vi "PyLoN_SRS3.vi"() -> ()   [LabVIEW 2014]
uses:
  Labview VIs/PIXIS_TEST/SITK_Labview/Examples70_2_2_0_1/RS Pixis/MaxY.vi
  Labview VIs/PIXIS_TEST/SITK_Labview/Examples70_2_2_0_1/RS Pixis/MaxX.vi
  <vilib>/Utility/file.llb/Write To Spreadsheet File (I64).vi
  <vilib>/Utility/file.llb/Write To Spreadsheet File (DBL).vi
panel:
  in  "stop":bool
  out "error out":errorcluster
  out "Description":string
  out "Increment":dbl
  out "Temperature 2":dbl=-75.0
  in  "error in":errorcluster
  out "x/y":dbl
  in  "CHEK ID":bool
  out "Max Value":dbl
  out "Min Value":dbl
  in  "Param ID":u32
  out "default value":dbl
  out "current value":dbl
  out "num of elements":dbl
  in  "?":bool
  in  "?":T1(tab)
  in  "Shutter State":u16(ring)=2 items=["Always Close", "Open Each Exposure", "Open Until Finish", "Open waiting for triger"]
  in  "Trigger Edge":u16(ring) items=["Positive", "Negative"]
  in  "Timing Mode":u16(ring) items=["Free Run", "Triger First", "Ext Sync", "Bulb Mode", "Variable Mode", "Flash Mode"]
  in  "ADC Speed":u16(ring)=2 items=["ADC Slowest", "ADC Fastest", "Default", "50 kHz", "100 kHz", "200 kHz", "500 kHz", "1 MHz"]
  in  "ADC Gain":u16(ring) items=["ADC Low", "ADC High"]
  in  "Temperature":dbl=-100.0 caption="SET Temperature" format="%.2f"
  in  "Skip Serial  Reg Clean":dbl=1.0 format="%.2f"
  in  "Vertical Timing":dbl=3.2
  out "Vertical Timing":dbl
  in  "Readout Port":i32=4 min=-1 step=1
  in  "?":T2={"X start"=0, "X end"=1023, "X Binning/Grouping"=1, "Y start"=0, "Y end"=1, "Y Binning/Grouping"=1}
  in  "Logic Out":u16(ring) items=["Not Scan", "Shutter", "Not Rady", "Logic 0", "Clearing", "Not Ft Image Shift", "Reserved", "Logic1", "Expos Prog", "Expos", "Image Shift", "Readout", "Acquiring", "Wait For Trig"]
  in  "Use Custom Timing":bool
  out "Readout Time":dbl caption="Readout time (ms)" format="%.2f"
  in  "Temp_bypass":bool
  in  "?":bool
  in  "Exposure Time (s)":dbl=0.004 min=0.0 step=0.001 format="%.3f"
  in  "?":bool
  in  "?":bool
  out "?":u16[](graph)
  in  "file path":path
  in  "File_name":string
  in  "# of spectrum per frame":i32
  in  "# of Frames":i32
  in  "FLIP SPECTRA":bool
  in  "?":bool
  in  "?":bool
  in  "?":bool
  out "?":dbl[](graph)
  in  "?":bool
  in  "Number of Images":u32=1 min=1 step=1
  out "?":dbl[](graph)
  in  "?":bool
  in  "# of Sets":i32
  out "Current Set":u32=24
  in  "#Ground per set":u32=3
  in  "Timepoints":dbl[](array[numeric])=[200.0, 100.0, 300.0, 400.0, 500.0]
  in  "File Path":path
  in  "File Name":string
  in  "Ground State\nSubstract?":bool
  in  "PyLonN Error In":errorcluster
  out "PyLoN Error Out":errorcluster
  out "PyLoN Ready":bool
  out "PyLoN \nTemperature":dbl
  # "REGION OF INTEREST"
  # "TRIGGER"
  # "ADC"
  # "SHUTTER"
  # "INPUT VARIABLES"
  # "TTL LOGIC"
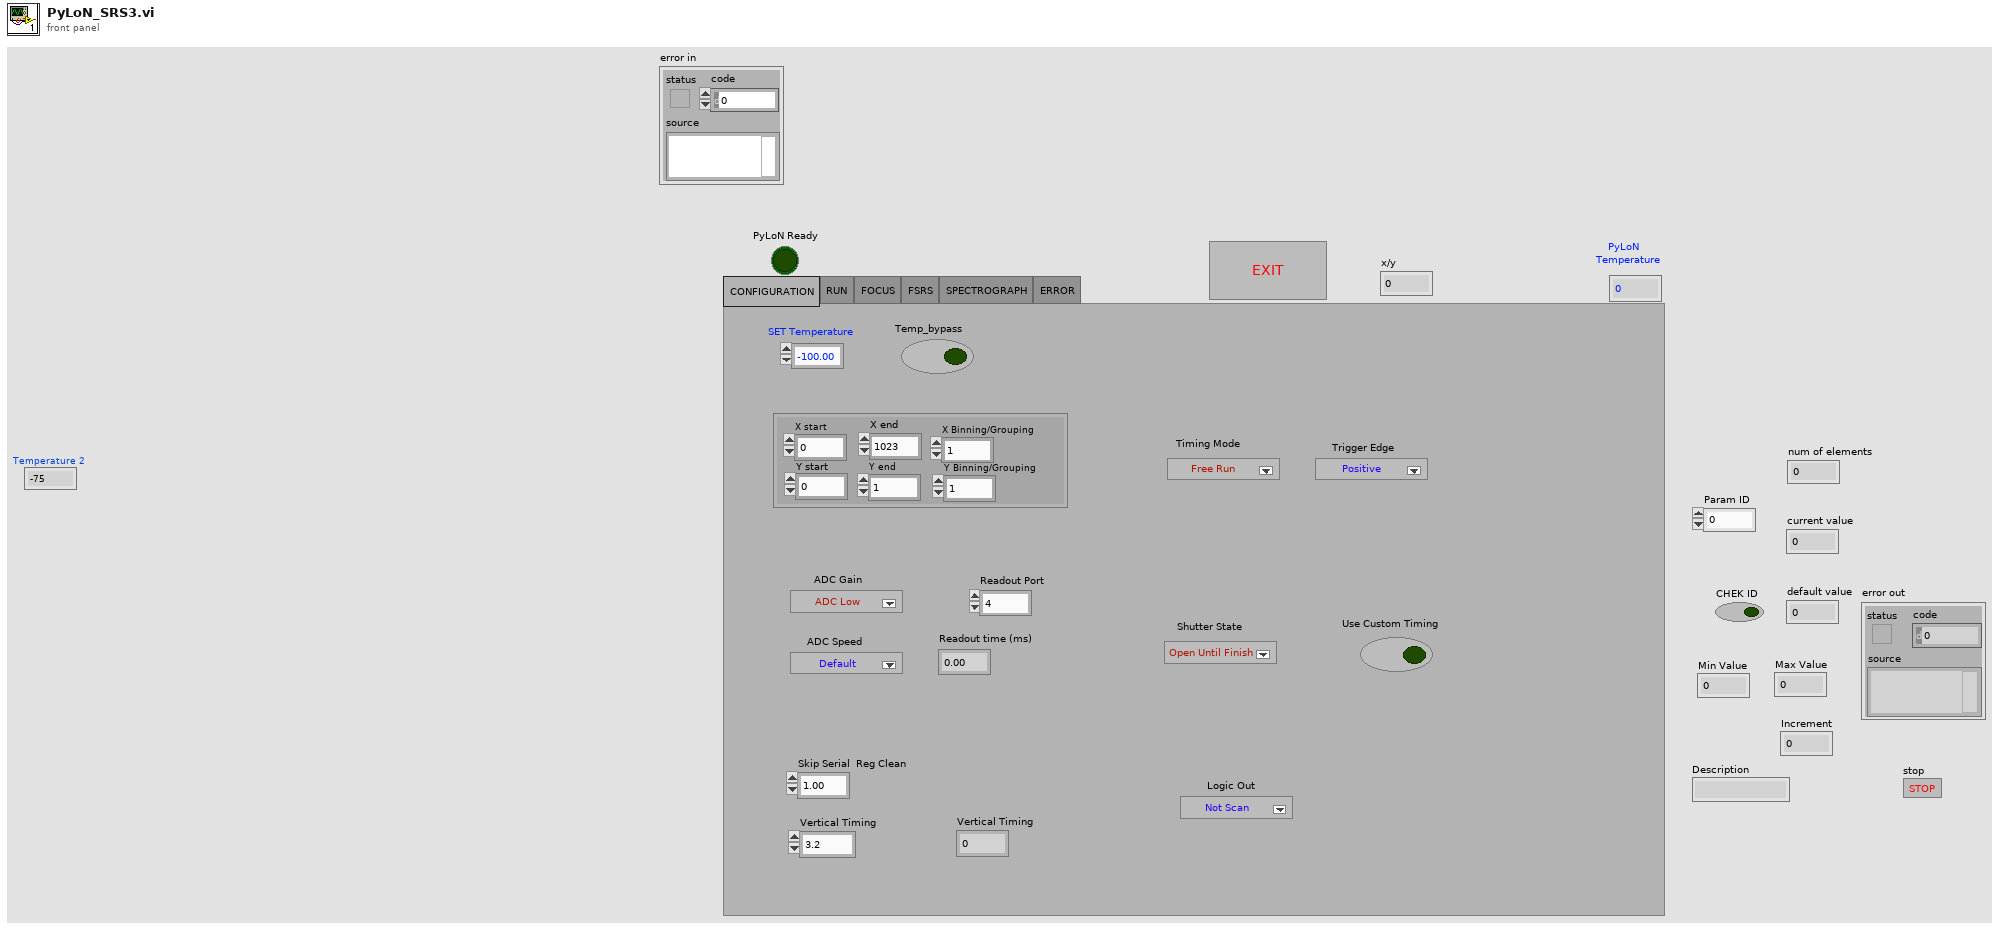
[diagram p1: front panel]
types:
  T1 = enum32{"CONFIGURATION", "RUN", "FOCUS", "FSRS", "SPECTROGRAPH", "ERROR"}
  T2 = cluster{"X start":u32, "X end":u32, "X Binning/Grouping":u32, "Y start":u32, "Y end":u32, "Y Binning/Grouping":u32}
  T3 = enum32{"Initializing", "RUN", "FSRS", "Monochromator", "Errors"}
  T4 = cluster{"Param ID":u32, "Avail Flag":u8, "Current Value":dbl, "Default Value":dbl, "Min Value":dbl, "Max Value":dbl, "Increment":dbl, "Data Type":u32, "Access Type":u32, "Bit Used Flag":u32, "Number of Enums":u32, "Description":string}
  T5 = cluster{"acquire focus mode":u32, "Exposure Time (s)":dbl, i32, "Software accumulation":u32}
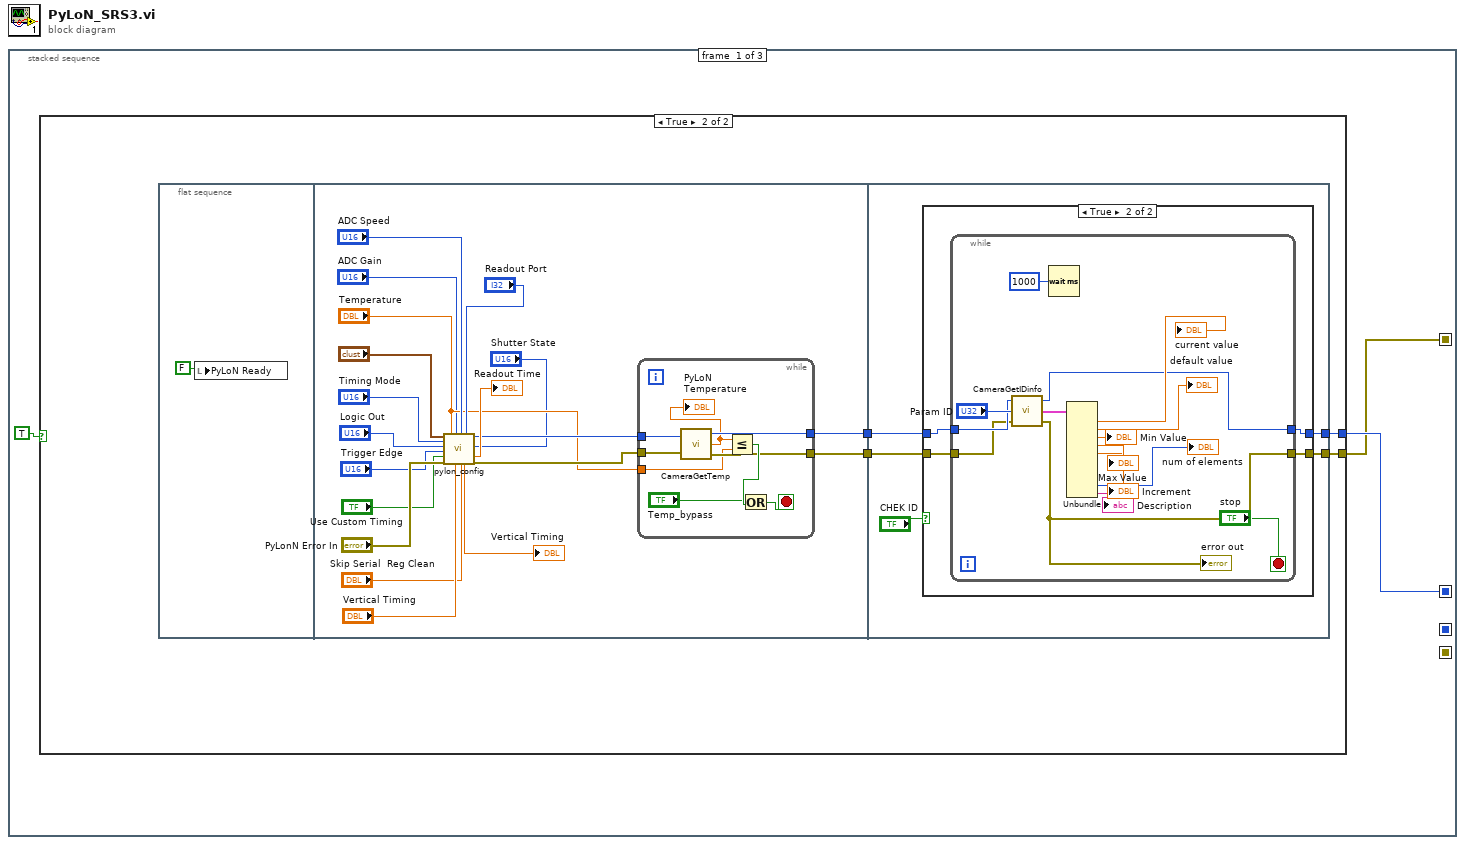
[diagram p0: block diagram]
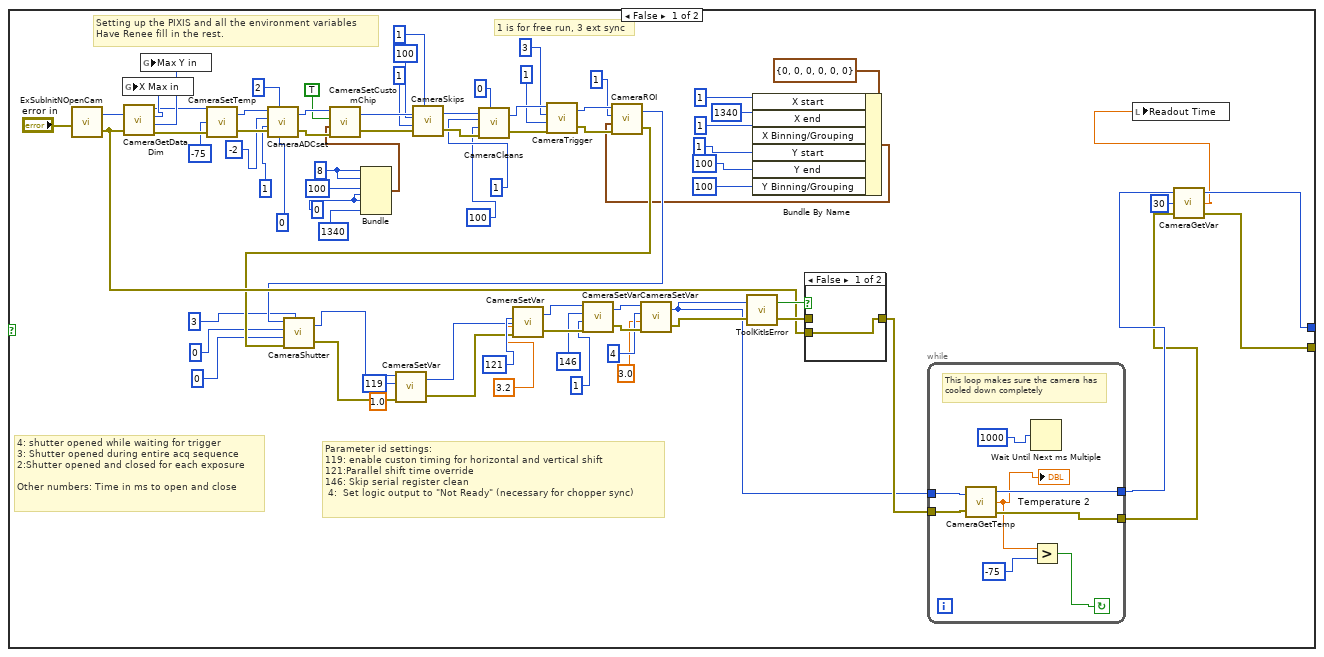
[diagram p2: hidden frame]
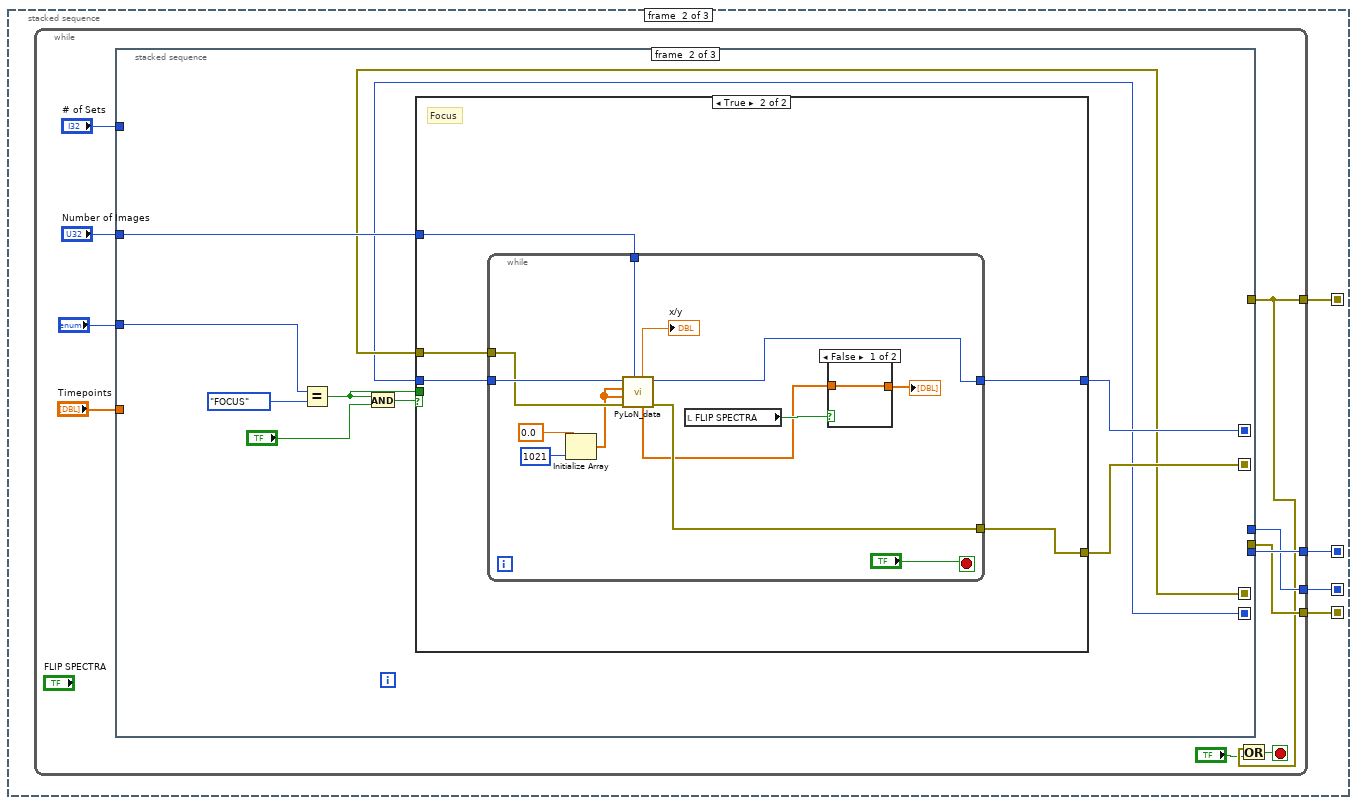
[diagram p5: hidden frame]
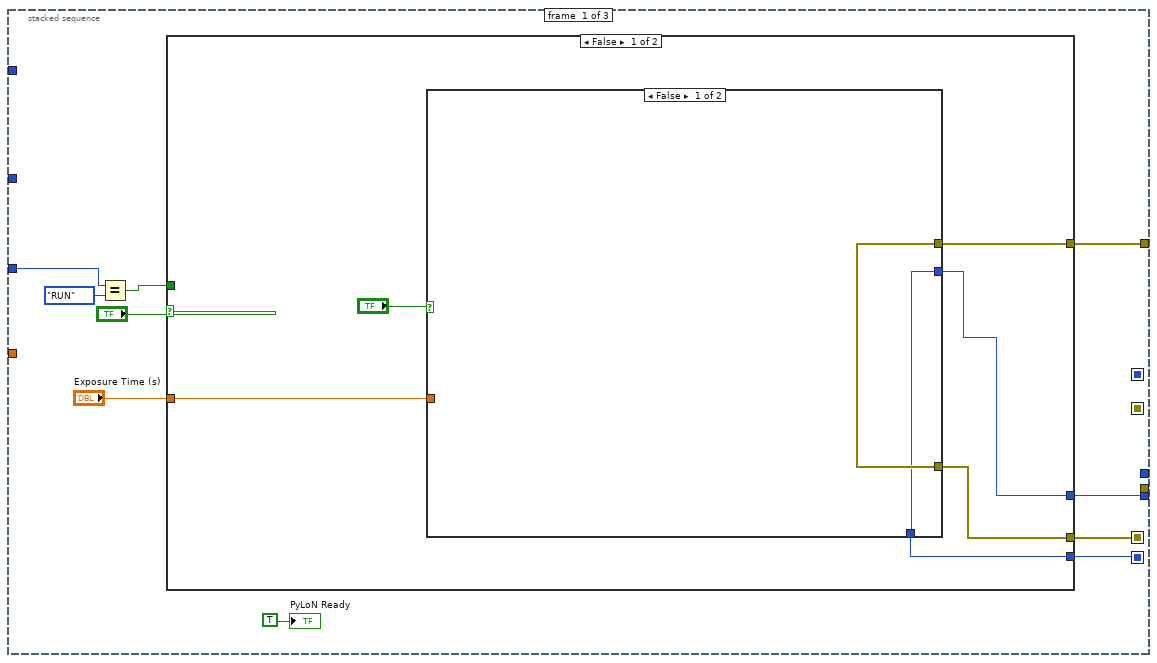
[diagram p6: hidden frame]
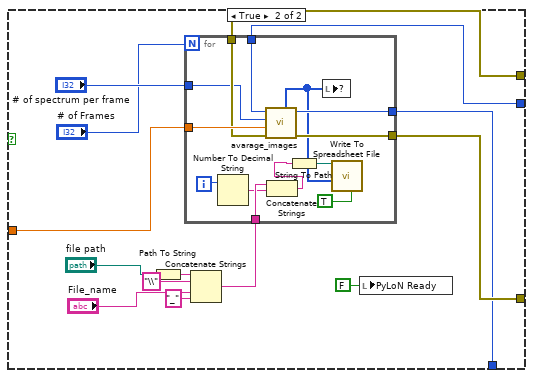
[diagram p7: hidden frame]
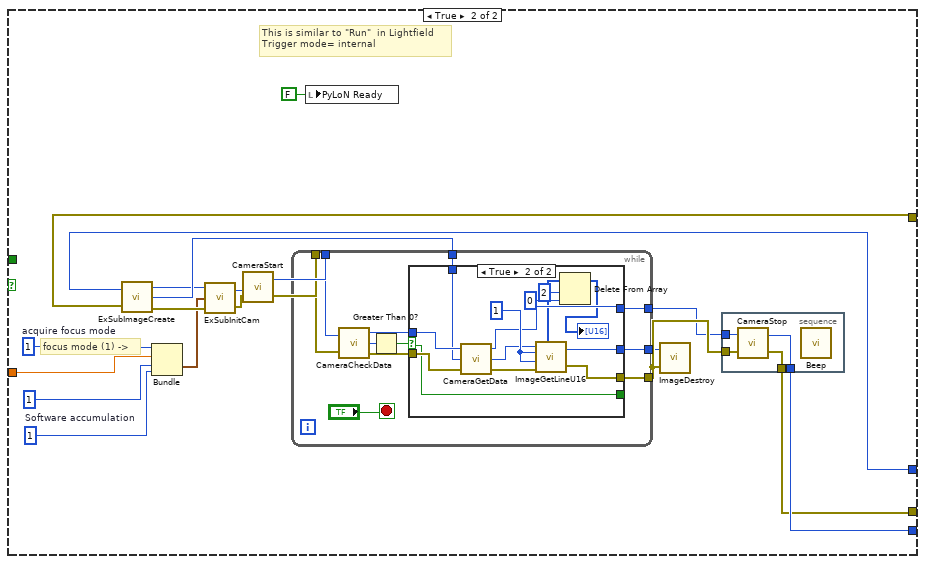
[diagram p8: hidden frame]
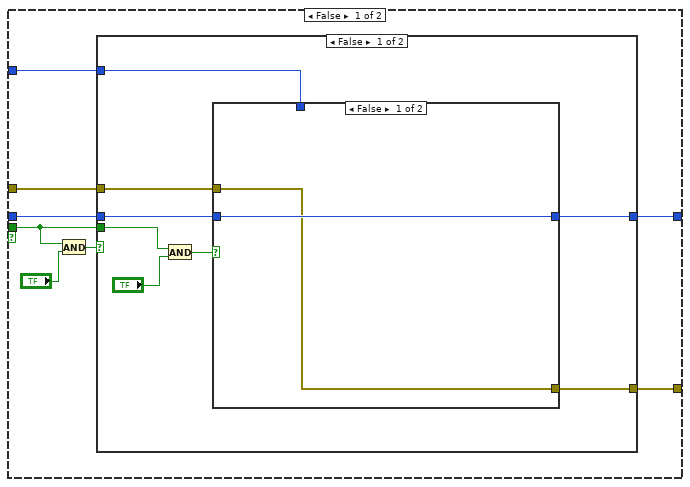
[diagram p10: hidden frame]
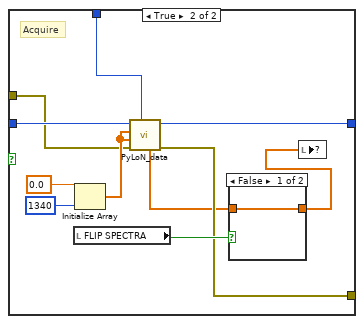
[diagram p11: hidden frame]
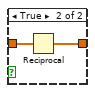
[diagram p12: hidden frame]
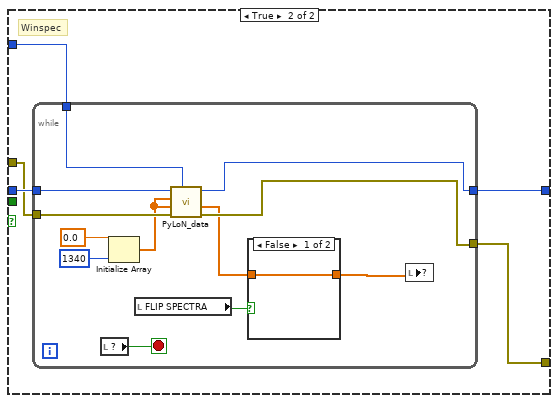
[diagram p13: hidden frame]
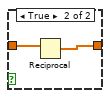
[diagram p14: hidden frame]
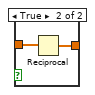
[diagram p15: hidden frame]
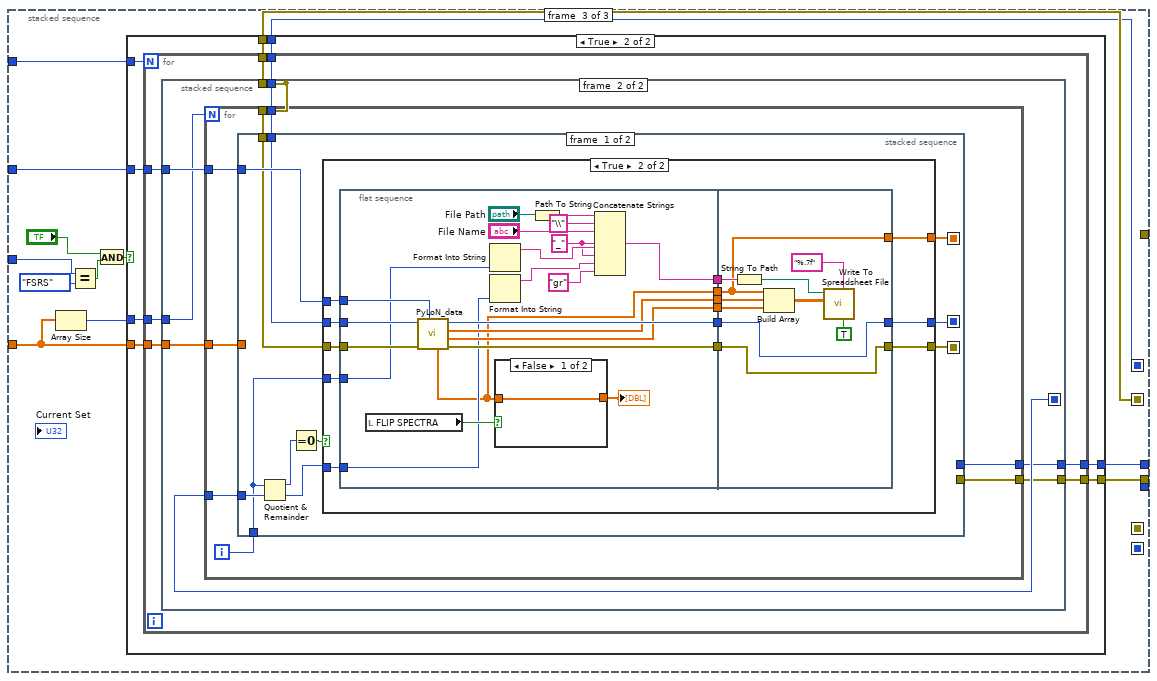
[diagram p16: hidden frame]
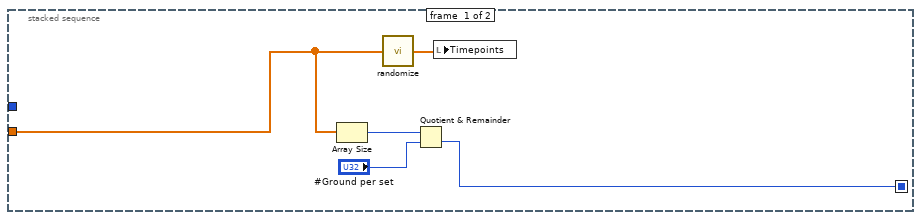
[diagram p18: hidden frame]
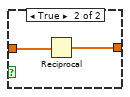
[diagram p20: hidden frame]
diagram:
  n1 = stacked-sequence {
    seq-local: [w1 _ _] -> [_ w152 _]
    seq-local: [w3 _ _] -> [_ w155 _]
    seq-local: [_ w154 _] -> [_ _ w517]
    seq-local: [_ w153 _] -> [_ _ w516]
    frame #0 {
      n2 = case shown="True" TRUE {
        tunnel: [w21 w94] -> w3
        tunnel: [w22 w93] -> w1
        frame False {
          w66 = 0
          w68 = 8
          # "4: shutter opened while waiting for trigger\n3: Shutter opened during entire acq sequence\n2:Shutter opened and closed for each exposure\n\nOther numbers: Time in ms to open and close"
          # "1 is for free run, 3 ext sync"
          # "Parameter id settings:\n119: enable custon timing for horizontal and vertical shift\n121:Parallel shift time override\n146: Skip serial register clean\n 4:  Set logic output to \"Not Ready\" (necessary for chopper sync)"
          # "Setting up the PIXIS and all the environment variables\nHave Renee fill in the rest."
          n3 = call "ExSubInitNOpenCam.vi"("error in (no error)"="error in") -> ("Camera Handle"=w81:u32, "error out"=w46:errorcluster)
          n4 = call <userlib>:"CameraGetDataDim.vi"("Camera Handle"=w81, "error in"=w46) -> ("Camera Handle"=w78:u32, "Xdim"=w80:u32, "Ydim"=w79:u32, "error out"=w77:errorcluster)
          n5 = global write "MaxX.vi" "X Max in"(w80) -> ()
          n6 = global write "MaxY.vi" "Max Y in"(w79) -> ()
          n7 = call <userlib>:"CameraSetTemp.vi"("error in (no error)"=w77, "Temperature"=-75, "Camera Handle"=w78) -> ("error out"=w74:errorcluster, "Camera Handle"=w75:u32)
          n8 = call <userlib>:"CameraADCset.vi"("ADC offset"=0, "Read Out port"=2, "error in (no error)"=w74, "ADC Gain"=1, "ADC Speed"=-2, "Camera Handle"=w75) -> ("error out"=w69:errorcluster, "Camera Handle"=w70:u32)
          n9 = Bundle(w68, w68, 100, w66, w66, 1340) -> (w64:cluster{i32, i32, i32, i32, i32, i32})  [unwired: 1 in]
          n10 = call <userlib>:"CameraSetCustomChip.vi"("error in (no error)"=w69, "Custom Chip Settings"=w64, "Enable/Disable Custom Chip"=TRUE, "Camera Handle"=w70) -> ("error out"=w61:errorcluster, "Camera Handle"=w62:u32)
          n11 = call <userlib>:"CameraSkips.vi"("Camera Handle"=w62, "Minimum Block Size"=100, "Number of Minimum blocks"=1, "error in"=w61, "Type of Skips"=1) -> ("Camera Handle"=w56:u32, "error out"=w57:errorcluster)
          n12 = call <userlib>:"CameraCleans.vi"("Camera Handle"=w56, "Number of Clears"=1, "Number of Strips Per Clear"=100, "error in"=w57, "Continuous Clears"=0) -> ("Camera Handle"=w51:u32, "error out"=w52:errorcluster)
          n13 = call <userlib>:"CameraTrigger.vi"("error in"=w52, "Trigger Edge"=1, "Timing Mode"=3, "Camera Handle"=w51) -> ("error out"=w38:errorcluster, "Camera Handle"=w37:u32)
          n14 = Bundle By Name(cluster=T2 {"X start"=0, "X end"=0, "X Binning/Grouping"=0, "Y start"=0, "Y end"=0, "Y Binning/Grouping"=0} ("ROI Params"), "X start"=u32 1, "X end"=u32 1340, "X Binning/Grouping"=u32 1, "Y start"=u32 1, "Y end"=u32 100, "Y Binning/Grouping"=u32 100) -> (w28:T2)
          n15 = call <userlib>:"CameraROI.vi"("error in"=w38, "ROI Params"=w28, "ROI Index"=1, "Camera Handle"=w37) -> ("error out"=w34:errorcluster, "Camera Handle"=w33:u32)
          n16 = call <userlib>:"CameraShutter.vi"("Camera Handle"=w33, "Shutter Comp Time: Pre Open"=0, "Shutter Comp Time: Post Open"=0, "error in"=w34, "Shutter State"=3) -> ("Camera Handle"=w9:u32, "error out"=w7:errorcluster)
          n17 = call <userlib>:"CameraSetVar.vi"("error in"=w7, "Value"=1.0, "Parameter ID"=u32 119, "Camera Handle"=w9) -> ("error out"=w6:errorcluster, "CameraHandle"=w8:u32)
          n18 = call <userlib>:"CameraSetVar.vi"("error in"=w6, "Value"=3.2, "Parameter ID"=121, "Camera Handle"=w8) -> ("error out"=w19:errorcluster, "CameraHandle"=w18:u32)
          n19 = call <userlib>:"CameraSetVar.vi"("error in"=w19, "Value"=1, "Parameter ID"=146, "Camera Handle"=w18) -> ("error out"=w14:errorcluster, "CameraHandle"=w13:u32)
          n20 = call <userlib>:"CameraSetVar.vi"("error in"=w14, "Value"=3.0, "Parameter ID"=4, "Camera Handle"=w13) -> ("error out"=w29:errorcluster, "CameraHandle"=w26:u32)
          n21 = call <userlib>:"ToolKitIsError.vi"("error in"=w29, "Reserved"=w26) -> ("error out"=w47:errorcluster, "Error Flag"=w48:bool)
          n22 = case shown="False" w48 {
            tunnel: w47 -> [_ w92]
            tunnel: [w91 w92] -> w27
            tunnel: w46 -> [w91 _]
            frame False {
            }
            frame True {
            }
          }
          n23 = while {
            tunnel: w27 -> [w89]
            tunnel: [w88] -> w23
            tunnel: w26 -> [w87]
            tunnel: [w86] -> w24
            stop <- w84 continue-if-true
            # "This loop makes sure the camera has cooled down completely"
            n24 = call <userlib>:"CameraGetTemp.vi"("Camera Handle"=w87, "error in (no error)"=w89) -> ("Camera Handle"=w86:u32, "Temperature"=w83:dbl, "error out"=w88:errorcluster)
            "Temperature 2" <- w83
            n25 = Wait Until Next ms Multiple(millisecond multiple=1000 ("ADC Gain")) -> ()  [unwired: 1 out]
            n26 = Greater?(x=w83, y=-75) -> (0:w84:bool)
          }
          n27 = call <userlib>:"CameraGetVar.vi"("error in"=w23, "Parameter ID"=u32 30, "Camera Handle"=w24) -> ("error out"=w22:errorcluster, "Value"=w20:dbl, "Camera Handle"=w21:u32)
          n28 = local write "Readout Time"(w20) -> ()
        }
        frame True {
          n29 = flat-sequence {
            tunnel: [w104] -> w96
            tunnel: [w102] -> w95
            tunnel: [w126] -> w93
            tunnel: [w129] -> w94
            tunnel: w96 -> [w130]
            tunnel: w95 -> [w128]
            frame #0 {
              n30 = local write "PyLoN Ready"(FALSE ("PyLoN Ready")) -> ()
            }
            frame #1 {
              n31 = call "pylon_config.vi"(0:"?", "Timing Mode"="Timing Mode", "Logic Out"="Logic Out", "Trigger Edge"="Trigger Edge", "Use Custom Chip"="Use Custom Timing", "PyLonN Error In"="PyLonN Error In", "Temperature"="Temperature", "ADC Gain"="ADC Gain", "Vertical Timing"="Vertical Timing", "ADC Speed"="ADC Speed", "Skip Serial  Reg Clean"="Skip Serial  Reg Clean", "Readout Port"="Readout Port", "Shutter State"="Shutter State") -> ("Vertical Timing"=→"Vertical Timing":dbl, "CameraHandle"=w105:u32, "Readout Time"=→"Readout Time":dbl, "error out"=w103:errorcluster)  [unwired: 3 in]
              n32 = while {
                tunnel: [w125] -> w104
                tunnel: w105 -> [w122]
                tunnel: w103 -> [w121]
                tunnel: [w120] -> w102
                tunnel: "Temperature" -> [w118]
                stop <- w124 stop-if-true
                n33 = call <userlib>:"CameraGetTemp.vi"("Camera Handle"=w122, "error in (no error)"=w121) -> ("Camera Handle"=w125:u32, "Temperature"=w119:dbl, "error out"=w120:errorcluster)
                "PyLoN \nTemperature" <- w119
                n34 = Less Or Equal?(x=w119, y=w118) -> (x <= y?=w123:bool)
                n35 = Or(x="Temp_bypass", y=w123) -> (x .or. y?=w124:bool)
              }
            }
            frame #2 {
              n36 = case shown="True" "CHEK ID" {
                tunnel: w130 -> [w132 w136]
                tunnel: [w132 w135] -> w129
                tunnel: w128 -> [w131 w134]
                tunnel: [w131 w133] -> w126
                frame False {
                }
                frame True {
                  n37 = while {
                    tunnel: w136 -> [w146]
                    tunnel: [w145] -> w135
                    tunnel: w134 -> [w144]
                    tunnel: [w143] -> w133
                    stop <- "stop" stop-if-true
                    n38 = call <userlib>:"CameraGetIDinfo.vi"("error in"=w144, "Param ID"="Param ID", "Camera handle"=w146) -> ("error out"=w143:errorcluster, "Param ID Information"=w151:T4, "Camera handle"=w145:u32)
                    "error out" <- w143
                    n39 = Wait (ms)(milliseconds to wait=u32 1000) -> ()  [unwired: 1 out]
                    n40 = Unbundle(w151) -> ("Current Value"=→"current value":dbl, "Default Value"=→"default value":dbl, "Min Value"=→"Min Value":dbl, "Max Value"=→"Max Value":dbl, "Increment"=→"Increment":dbl, "Number of Enums"=→"num of elements":u32, "Description"=→"Description":string)  [unwired: 5 out]
                  }
                }
              }
            }
          }
        }
      }
    }
    frame #1 {
      n41 = while {
        tunnel: w155 -> [w165]
        tunnel: w152 -> [w157]
        tunnel: [w161] -> w154
        tunnel: [w160] -> w153
        stop <- w158 stop-if-true
        n42 = stacked-sequence {
          seq-local: [_ w268 _] -> [_ _ w353]
          seq-local: [_ w267 _] -> [_ _ w355]
          seq-local: [w170 _ _] -> [_ w265 _]
          seq-local: [w171 _ _] -> [_ w266 _]
          tunnel: w165 -> [w168 _ _]
          tunnel: w157 -> [w175 _ _]
          tunnel: "?" -> [w172 w273 w359]
          tunnel: "Number of Images" -> [_ w271 w356]
          tunnel: "Timepoints" -> [_ _ w348]
          tunnel: [_ _ w352] -> w161
          tunnel: [_ _ w351] -> w160
          tunnel: "# of Sets" -> [_ _ w349]
          frame #0 {
            n43 = Equal?(x=w172, y=T3."RUN") -> (x = y?=w169:bool)
            n44 = case shown="False" "?" {
              tunnel: w175 -> [w181 w213]
              tunnel: [w178 w216] -> w170
              tunnel: [w180 w215] -> w171
              tunnel: w169 -> [_ _]
              tunnel: w168 -> [w179 w214]
              tunnel: "Exposure Time (s)" -> [w177 w211]
              frame False {
                n45 = case shown="False" "?" {
                  tunnel: w181 -> [w183 w195]
                  tunnel: [w183 w194] -> w180
                  tunnel: w179 -> [w182 w196]
                  tunnel: [w182 w193] -> w178
                  tunnel: w177 -> [_ w197]
                  frame False {
                  }
                  frame True {
                    n46 = Path To String(path="file path") -> (string=w189:string)
                    n47 = Concatenate Strings(w189, "\\" ("string"), "File_name", "_" ("string")) -> (w184:string)
                    n48 = for {
                      N: "# of Frames" -> [_]
                      tunnel: w197 -> [w210]
                      tunnel: w196 -> [w209]
                      tunnel: w195 -> [w208]
                      tunnel: [w207] -> w194
                      tunnel: [w206] -> w193
                      tunnel: "# of spectrum per frame" -> [w205]
                      tunnel: w184 -> [w201]
                      i -> [w198]
                      n49 = Number To Decimal String(number=w198) -> (decimal integer string=w200:string)  [unwired: 1 in]
                      n50 = call "avarage_images.vi"("error in (no error)"=w208, "Exposure Time (s)"=w210, "Number of Images"=w205, "Camera Handle"=w209) -> ("error out"=w207:errorcluster, "Camera Handle"=w206:u32, "Waveform Graph"=w204:i32[])  [unwired: 3 in, 2 out]
                      n51 = Concatenate Strings(w201, w200) -> (w199:string)
                      n52 = String To Path(string=w199) -> (path=w202:path)
                      n53 = local write item#9(w204) -> ()
                      n54 = call-poly <vilib>:"Write To Spreadsheet File.vi"("transpose? (no:F)"=TRUE, "1D data"=w204, "file path (dialog if empty)"=w202) -> ()  [unwired: 5 in, 1 out]
                    }
                    n55 = local write "PyLoN Ready"(FALSE ("PyLoN Ready")) -> ()
                  }
                }
              }
              frame True {
                w218 = u32 1  # acquire focus mode
                w219 = u32 1  # Software accumulation
                # "focus mode (1) ->"
                # "This is similar to \"Run\"  in Lightfield\nTrigger mode= internal"
                n56 = call "ExSubImageCreate.vi"("Camera Handle"=w214, "error in (no error)"=w213) -> ("Camera Handle"=w220:u32, "Data Handle"=w226:u32, "error out"=w221:errorcluster)
                n57 = Bundle("acquire focus mode"=w218, "Exposure Time (s)"=w211, 1, "Software accumulation"=w219) -> (w217:T5)  [unwired: 1 in]
                n58 = call "ExSubInitCam.vi"("error in (no error)"=w221, "Camera Information"=w217, "Camera Handle"=w220) -> ("error out"=w222:errorcluster, "Camera Handle"=w223:u32)
                n59 = call <userlib>:"CameraStart.vi"("error in"=w222, "Camera Handle"=w223) -> ("error out"=w224:errorcluster, "Camera Handle"=w225:u32)
                n60 = while {
                  tunnel: [w241] -> w227
                  tunnel: [w240] -> w229
                  tunnel: [w239] -> w228
                  tunnel: w224 -> [w238]
                  tunnel: w225 -> [w237]
                  tunnel: w226 -> [w236]
                  stop <- "?" stop-if-true
                  n61 = call <userlib>:"CameraCheckData.vi"("Camera Handle"=w237, "error in"=w238) -> ("Camera Handle"=w243:u32, "Number Of Frames Available"=w245:i32, "error out"=w242:errorcluster)
                  n62 = Greater Than 0?(x=w245) -> (x > 0?=w244:bool)
                  n63 = case shown="True" w244 {
                    selector: w244 -> [w248 w261]
                    tunnel: w243 -> [w246 w263]
                    tunnel: w242 -> [w249 w262]
                    tunnel: [w248 w261] -> _
                    tunnel: [w249 w260] -> w240
                    tunnel: w236 -> [w247 w254]
                    tunnel: [w247 w258] -> w241
                    tunnel: [w246 w257] -> w239
                    frame False {
                    }
                    frame True {
                      w259 = 1
                      n64 = call <userlib>:"CameraGetData.vi"("error in"=w262, "Image/Data Handle"=w254, "Camera Handle"=w263) -> ("error out"=w256:errorcluster, "Image/Data Handle"=w255:u32, "Camera Handle"=w257:u32)
                      n65 = call <userlib>:"ImageGetLineU16.vi"("Data Handle"=w255, "Y Position"=w259, "Z Position"=w259, "error in"=w256) -> ("Array u16"=w253:u16[], "Data Handle"=w258:u32, "error out"=w260:errorcluster)
                      n66 = Delete From Array(array=w253, length=2, index=0) -> (array with subset deleted=→"?":u16[])  [unwired: 1 out]
                    }
                  }
                }
                n67 = local write "PyLoN Ready"(FALSE ("PyLoN Ready")) -> ()
                n68 = call <userlib>:"ImageDestroy.vi"("error in"=w229, "Data handle"=w227) -> ()  [unwired: 1 out]
                n69 = stacked-sequence {
                  tunnel: w229 -> [w234]
                  tunnel: w228 -> [w233]
                  tunnel: [w232] -> w215
                  tunnel: [w231] -> w216
                  frame #0 {
                    n70 = call <userlib>:"CameraStop.vi"("error in"=w234, "Camera Handle"=w233) -> ("error out"=w232:errorcluster, "Camera Handle"=w231:u32)
                    n71 = call <vilib>:"Beep.vi"() -> ()  [unwired: 12 in]
                  }
                }
              }
            }
            "PyLoN Ready" <- TRUE
          }
          frame #1 {
            n72 = Equal?(x=w273, y=T1."FOCUS") -> (x = y?=w269:bool)
            n73 = And(x=w269, y="?") -> (x .and. y?=w272:bool)
            n74 = case shown="True" w272 {
              tunnel: w265 -> [w281 w330]
              tunnel: [w277 w329] -> w268
              tunnel: w266 -> [w279 w328]
              tunnel: w271 -> [w280 w327]
              tunnel: [w278 w326] -> w267
              tunnel: w269 -> [w274 _]
              frame False {
                n75 = And(x=w274, y="?") -> (x .and. y?=w276:bool)
                n76 = case shown="False" w276 {
                  tunnel: w281 -> [w284 w310]
                  tunnel: w280 -> [w285 w309]
                  tunnel: w279 -> [w286 w308]
                  tunnel: [w282 w307] -> w278
                  tunnel: [w283 w306] -> w277
                  tunnel: w274 -> [w287 _]
                  frame False {
                    n77 = And(x=w287, y="?") -> (x .and. y?=w289:bool)
                    n78 = case shown="False" w289 {
                      tunnel: w286 -> [w290 w295]
                      tunnel: w285 -> [_ w298]
                      tunnel: w284 -> [w291 w297]
                      tunnel: [w291 w293] -> w283
                      tunnel: [w290 w294] -> w282
                      frame False {
                      }
                      frame True {
                        # "Acquire"
                        n79 = local read "FLIP SPECTRA"() -> (w300:bool)
                        n80 = Initialize Array(0.0, u32 1340) -> (w296:dbl[])
                        n81 = call "PyLoN_data.vi"("Number of Images"=w298, "error in (no error)"=w295, "PumpOffBkgd"=w296, "PumpOnBkgd"=w296, "Camera Handle"=w297) -> ("error out"=w294:errorcluster, "Camera Handle 2"=w293:u32, "Raman_Gain"=w292:dbl[])  [unwired: 1 in, 3 out]
                        n82 = case shown="False" w300 {
                          tunnel: w292 -> [w303 w305]
                          tunnel: [w303 w304] -> w299
                          frame False {
                          }
                          frame True {
                            n83 = Reciprocal(x=w305) -> (1/x=w304:dbl[])
                          }
                        }
                        n84 = local write item#21(w299) -> ()
                      }
                    }
                  }
                  frame True {
                    # "Winspec"
                    n85 = while {
                      tunnel: w310 -> [w316]
                      tunnel: w309 -> [w317]
                      tunnel: [w311] -> w306
                      tunnel: w308 -> [w315]
                      tunnel: [w314] -> w307
                      stop <- w320 stop-if-true
                      n86 = local read item#27() -> (w320:bool)
                      n87 = Initialize Array(0.0, u32 1340) -> (w312:dbl[])
                      n88 = local read "FLIP SPECTRA"() -> (w319:bool)
                      n89 = call "PyLoN_data.vi"("Number of Images"=w317, "error in (no error)"=w315, "PumpOffBkgd"=w312, "PumpOnBkgd"=w312, "Camera Handle"=w316) -> ("error out"=w314:errorcluster, "Pump_Off"=w313:dbl[], "Camera Handle 2"=w311:u32)  [unwired: 1 in, 3 out]
                      n90 = case shown="False" w319 {
                        tunnel: w313 -> [w323 w324]
                        tunnel: [w323 w325] -> w318
                        frame False {
                        }
                        frame True {
                          n91 = Reciprocal(x=w324) -> (1/x=w325:dbl[])
                        }
                      }
                      n92 = local write item#21(w318) -> ()
                    }
                  }
                }
              }
              frame True {
                # "Focus"
                n93 = while {
                  tunnel: w328 -> [w336]
                  tunnel: w327 -> [w337]
                  tunnel: [w335] -> w326
                  tunnel: w330 -> [w338]
                  tunnel: [w333] -> w329
                  stop <- "?" stop-if-true
                  n94 = Initialize Array(0.0, u32 1021) -> (w334:dbl[])
                  n95 = call "PyLoN_data.vi"("Number of Images"=w337, "error in (no error)"=w336, "PumpOffBkgd"=w334, "PumpOnBkgd"=w334, "Camera Handle"=w338) -> ("error out"=w335:errorcluster, "Camera Handle 2"=w333:u32, "Raman_Gain"=w332:dbl[], "x/y"=→"x/y":dbl)  [unwired: 1 in, 2 out]
                  n96 = local read "FLIP SPECTRA"() -> (w340:bool)
                  n97 = case shown="False" w340 {
                    tunnel: w332 -> [w344 w346]
                    tunnel: [w344 w345] -> w339
                    frame False {
                    }
                    frame True {
                      n98 = Reciprocal(x=w346) -> (1/x=w345:dbl[])
                    }
                  }
                  "?" <- w339
                }
              }
            }
          }
          frame #2 {
            n99 = Array Size(array=w348) -> (size(s)=w347:i32)
            n100 = Equal?(x=w359, y=T1."FSRS") -> (x = y?=w357:bool)
            n101 = And(x="?", y=w357) -> (x .and. y?=w358:bool)
            n102 = case shown="True" w358 {
              tunnel: w356 -> [_ w369]
              tunnel: w353 -> [w360 w368]
              tunnel: w355 -> [w361 w364]
              tunnel: w348 -> [_ w367]
              tunnel: [w360 w366] -> w352
              tunnel: [w361 w365] -> w351
              tunnel: w349 -> [_ w363]
              tunnel: w347 -> [_ w362]
              frame False {
              }
              frame True {
                n103 = for {
                  N: w363 -> [_]
                  tunnel: w369 -> [w376]
                  tunnel: w368 -> [w375]
                  tunnel: w367 -> [w374]
                  tunnel: [w373] -> w366
                  tunnel: [w372] -> w365
                  tunnel: w364 -> [w371]
                  tunnel: w362 -> [w370]
                  n104 = stacked-sequence {
                    seq-local: [w379 _] -> [_ w389]
                    tunnel: w376 -> [_ w388]
                    tunnel: w375 -> [_ w387]
                    tunnel: [_ w383] -> _
                    tunnel: w374 -> [w377 w386]
                    tunnel: [_ w385] -> w372
                    tunnel: [_ w384] -> w373
                    tunnel: w371 -> [_ w383]
                    tunnel: w370 -> [_ w382]
                    frame #0 {
                      n105 = Array Size(array=w377) -> (size(s)=w381:i32)
                      n106 = call "randomize.vi"("Input array"=w377) -> ("Output array"=w378:dbl[])
                      n107 = Quotient & Remainder(x=w381, y="#Ground per set") -> (floor(x/y)=w379:u32)  [unwired: 1 out]
                      n108 = local write "Timepoints"(w378) -> ()
                    }
                    frame #1 {
                      n109 = for {
                        N: w382 -> [_]
                        tunnel: w389 -> [w396]
                        tunnel: w388 -> [w395]
                        tunnel: w387 -> [w394]
                        tunnel: w386 -> [w393]
                        tunnel: [w392] -> w385
                        tunnel: [w391] -> w384
                        tunnel: w383 -> [w390]
                        i -> [w397]
                        n110 = stacked-sequence {
                          seq-local: [w399 _] -> [_ w462]
                          seq-local: [w400 _] -> [_ w463]
                          seq-local: [w398 _] -> [_ w461]
                          tunnel: w397 -> [w401 w464]
                          tunnel: w396 -> [w406 _]
                          tunnel: w395 -> [w404 w466]
                          tunnel: w394 -> [w403 _]
                          tunnel: w390 -> [w402 _]
                          tunnel: w393 -> [_ w465]
                          tunnel: [_ w460] -> w392
                          tunnel: [_ w459] -> w391
                          frame #0 {
                            n111 = Quotient & Remainder(x=w401, y=w406) -> (x-y*floor(x/y)=w407:u32, floor(x/y)=w405:u32)
                            n112 = Equal To 0?(x=w407) -> (x = 0?=w408:bool)
                            n113 = case shown="True" w408 {
                              tunnel: w405 -> [_ w420]
                              tunnel: w404 -> [_ w424]
                              tunnel: w403 -> [w410 w423]
                              tunnel: w402 -> [w409 w422]
                              tunnel: [w410 w413] -> w399
                              tunnel: [w409 w412] -> w400
                              tunnel: w401 -> [_ w421]
                              tunnel: [_ w411] -> w398
                              frame False {
                              }
                              frame True {
                                n114 = flat-sequence {
                                tunnel: w424 -> [w445]
                                tunnel: w423 -> [w444]
                                tunnel: w422 -> [w443]
                                tunnel: w421 -> [w431]
                                tunnel: w420 -> [w429]
                                tunnel: [w442] -> w419
                                tunnel: [w441] -> w418
                                tunnel: [w438] -> w417
                                tunnel: [w437] -> w416
                                tunnel: [w426] -> w415
                                tunnel: [w425] -> w414
                                tunnel: w419 -> [w451]
                                tunnel: w418 -> [w450]
                                tunnel: w417 -> [w454]
                                tunnel: w416 -> [w453]
                                tunnel: w415 -> [w455]
                                tunnel: w414 -> [w449]
                                tunnel: [w451] -> w413
                                tunnel: [w450] -> w412
                                tunnel: [w449] -> w411
                                frame #0 {
                                w430 = "_" ("string")
                                n115 = local read "FLIP SPECTRA"() -> (w440:bool)
                                n116 = call "PyLoN_data.vi"("Number of Images"=w445, "error in (no error)"=w443, "Camera Handle"=w444) -> ("error out"=w441:errorcluster, "Pump_Off"=w437:dbl[], "Pump_On"=w438:dbl[], "Camera Handle 2"=w442:u32, "Raman_Gain"=w425:dbl[])  [unwired: 3 in, 1 out]
                                n117 = Format Into String(w431) -> (resulting string=w432:string)  [unwired: 3 in, 1 out]
                                n118 = Format Into String(w429) -> (resulting string=w428:string)  [unwired: 3 in, 1 out]
                                n119 = case shown="False" w440 {
                                tunnel: w425 -> [w446 w448]
                                tunnel: [w446 w447] -> w439
                                frame False {
                                }
                                frame True {
                                n120 = Reciprocal(x=w448) -> (1/x=w447:dbl[])
                                }
                                }
                                "?" <- w439
                                n121 = Path To String(path="File Path") -> (string=w436:string)
                                n122 = Concatenate Strings(w436, "\\" ("string"), "File Name", w430, w432, w430, w428, "gr" ("string")) -> (w426:string)
                                }
                                frame #1 {
                                n123 = String To Path(string=w455) -> (path=w456:path)
                                n124 = Build Array(w449, w454, w453) -> (w452:dbl[][])
                                n125 = call-poly <vilib>:"Write To Spreadsheet File.vi"("transpose? (no:F)"=TRUE, "format (%.3f)"="%.7f", "2D data"=w452, "file path (dialog if empty)"=w456) -> ()  [unwired: 4 in, 1 out]
                                }
                                }
                              }
                            }
                          }
                          frame #1 {
                            n126 = stacked-sequence {
                              seq-local: [_ w469 _ _ _] -> [_ _ _ w490 _]
                              seq-local: [_ w472 _ _ _] -> [_ _ _ w489 w496]
                              seq-local: [_ w471 _ _ _] -> [_ _ _ w488 _]
                              seq-local: [_ w470 _ _ _] -> [_ _ _ w487 _]
                              tunnel: w463 -> [_ w482 _ _ _]
                              tunnel: w462 -> [_ w481 _ _ _]
                              tunnel: w466 -> [_ w480 _ _ _]
                              tunnel: w465 -> [_ w477 _ _ _]
                              tunnel: w464 -> [_ w473 _ _ _]
                              tunnel: w461 -> [_ _ _ _ w497]
                              tunnel: [_ w468 _ _ _] -> w460
                              tunnel: [_ w467 _ _ _] -> w459
                              frame #0 {
                              }
                              frame #1 {
                                n127 = Index Array(array=w477, index=w473) -> (element=w476:dbl)
                                n128 = call "tppathcr.vi"("input"=w476) -> ("out"=w475:string)
                                n129 = local read "File Path"() -> (w479:path)
                                n130 = local read "File Name"() -> (w478:string)
                                n131 = call "PyLoN_data.vi"("Number of Images"=w480, "error in (no error)"=w482, "Camera Handle"=w481) -> ("error out"=w468:errorcluster, "Pump_Off"=w470:dbl[], "Pump_On"=w471:dbl[], "Camera Handle 2"=w467:u32, "Raman_Gain"=w472:dbl[])  [unwired: 3 in, 1 out]
                                n132 = Format Into String(w473) -> (resulting string=w483:string)  [unwired: 3 in, 1 out]
                                n133 = Path To String(path=w479) -> (string=w486:string)
                                n134 = Concatenate Strings(w486, "\\" ("string"), w478, "_" ("string"), w475, "exe" ("string"), w483) -> (w469:string)
                              }
                              frame #2 {
                              }
                              frame #3 {
                                n135 = String To Path(string=w490) -> (path=w492:path)
                                n136 = Build Array(w489, w488, w487) -> (w491:dbl[][])
                                n137 = call-poly <vilib>:"Write To Spreadsheet File.vi"("transpose? (no:F)"=TRUE, "format (%.3f)"="%.7f", "2D data"=w491, "file path (dialog if empty)"=w492) -> ()  [unwired: 4 in, 1 out]
                              }
                              frame #4 {
                                n138 = case shown="False" "Ground State\nSubstract?" {
                                tunnel: w497 -> [_ w506]
                                tunnel: w496 -> [w500 w505]
                                frame False {
                                n139 = local read "FLIP SPECTRA"() -> (w499:bool)
                                n140 = case shown="True" w499 {
                                tunnel: [w501 w503] -> w498
                                tunnel: w500 -> [w501 w502]
                                frame False {
                                }
                                frame True {
                                n141 = Reciprocal(x=w502) -> (1/x=w503:dbl[])
                                }
                                }
                                n142 = local write item#33(w498) -> ()
                                }
                                frame True {
                                n143 = local read "FLIP SPECTRA"() -> (w507:bool)
                                n144 = case shown="False" w507 {
                                tunnel: [w510 w515] -> w509
                                tunnel: w506 -> [w511 w512]
                                tunnel: [w511 w514] -> w508
                                tunnel: w505 -> [w510 w513]
                                frame False {
                                }
                                frame True {
                                n145 = Reciprocal(x=w513) -> (1/x=w515:dbl[])
                                n146 = Reciprocal(x=w512) -> (1/x=w514:dbl[])
                                }
                                }
                                n147 = Subtract(x=w509, y=w508) -> (x-y=w504:dbl[])
                                n148 = local write item#33(w504) -> ()
                                }
                                }
                              }
                            }
                          }
                        }
                      }
                    }
                  }
                }
              }
            }
          }
        }
        n149 = Or(x=w157, y="?") -> (x .or. y?=w158:bool)
      }
    }
    frame #2 {
      n150 = local write "PyLoN Ready"(FALSE ("PyLoN Ready")) -> ()
      n151 = call "ExSubCloseCamUnInit.vi"("error in (no error)"=w516, "Camera Handle"=w517) -> ("error out"=→"PyLoN Error Out":errorcluster)
    }
  }
